vi "8742.vi"() -> ()   [LabVIEW 2012]
panel:
  out "Axis4 Mov":bool
  out "Axis3 Mov":bool
  out "Axis2 Mov":bool
  out "Axis1 Mov":bool
  out "Axis4 Pos":dbl
  out "Axis3 Pos":dbl
  out "Axis2 Pos":dbl
  out "Axis1 Pos":dbl
  in  "Axis4 set":dbl
  in  "Axis3 set":dbl
  in  "Axis2 set":dbl
  in  "Axis1 set":dbl
  in  "停止":bool
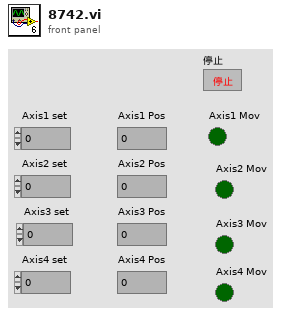
[diagram p1: front panel]
types:
  T1 = cluster{"CmdLib Out":refnum<k24>, "DeviceKey Out":string, "Device Address":i32}
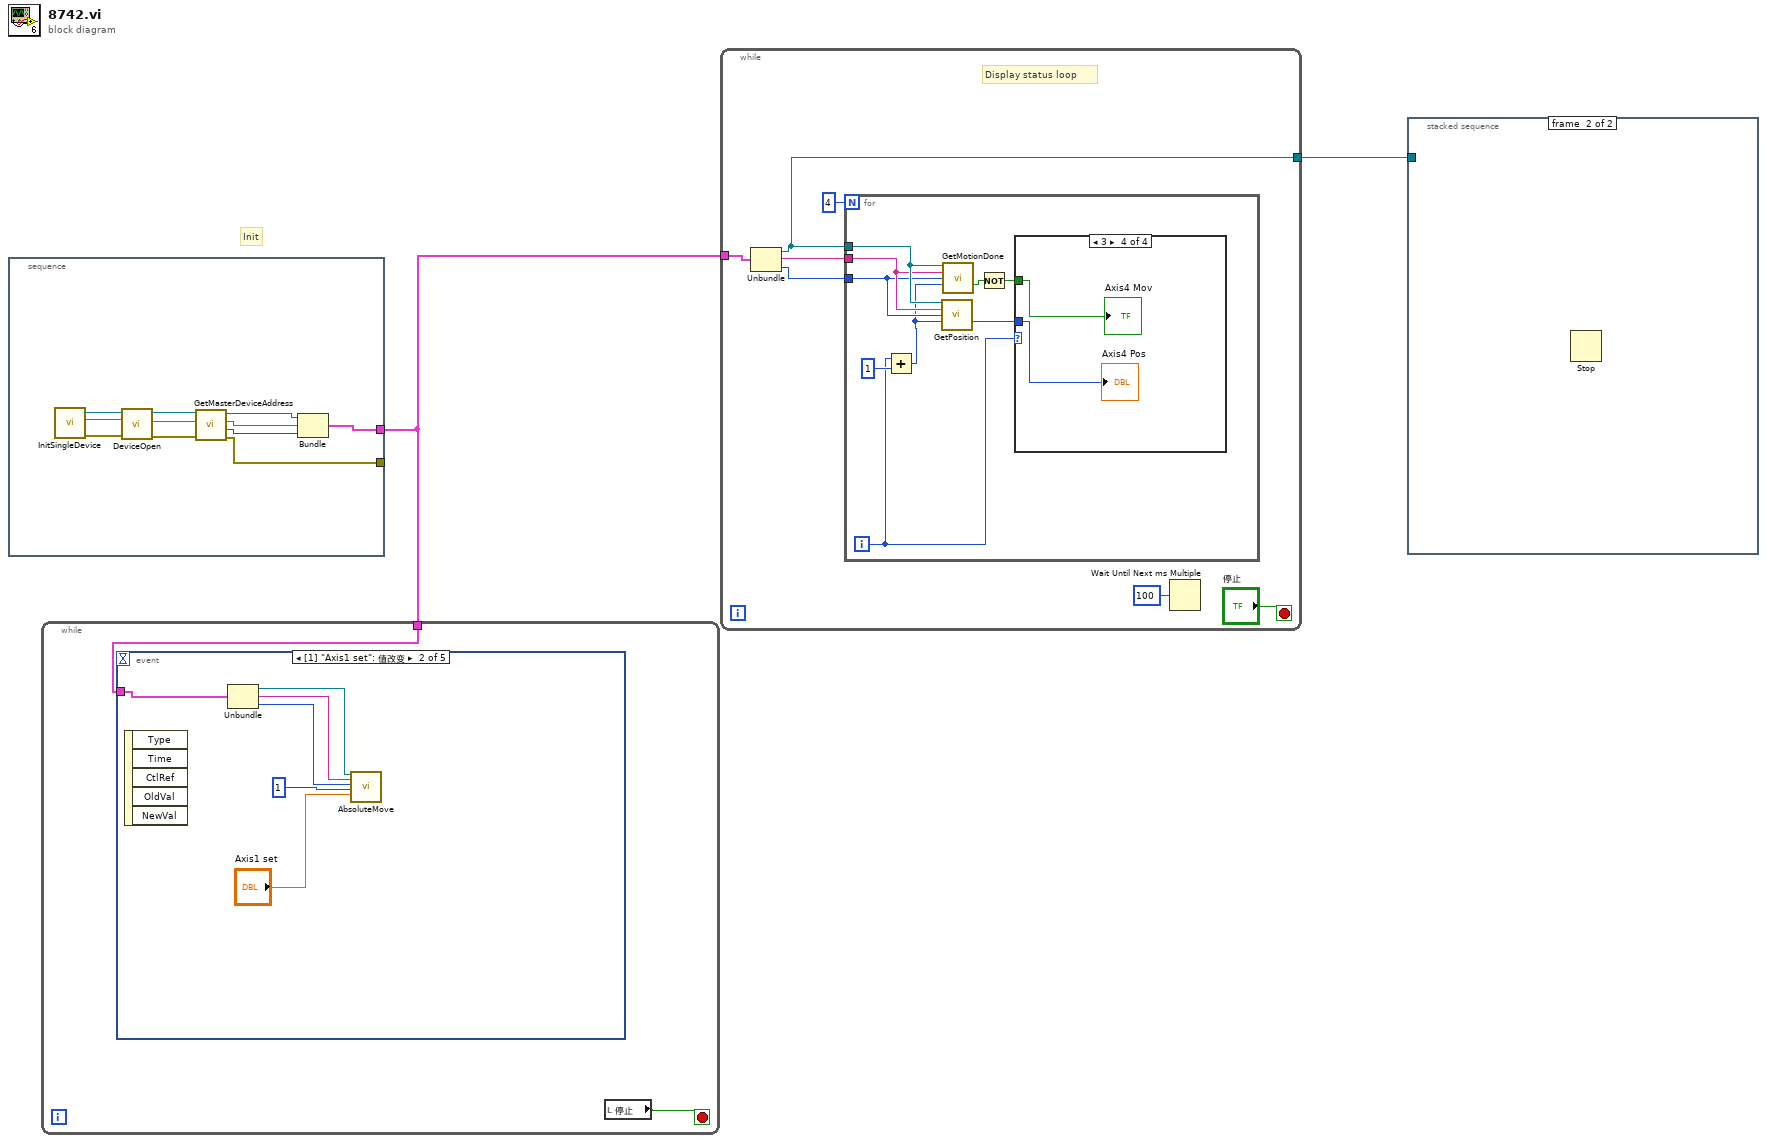
[diagram p0: block diagram]
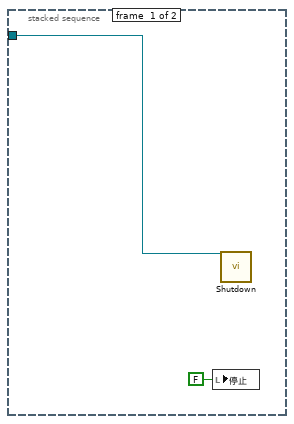
[diagram p2: hidden frame]
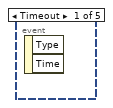
[diagram p3: hidden frame]
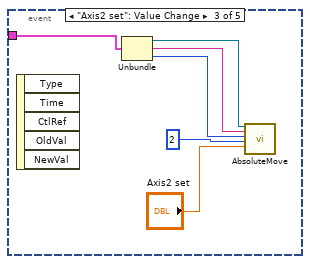
[diagram p4: hidden frame]
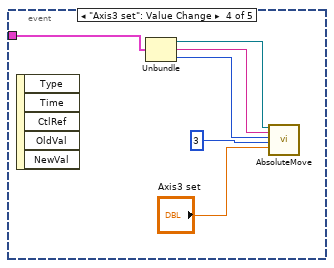
[diagram p5: hidden frame]
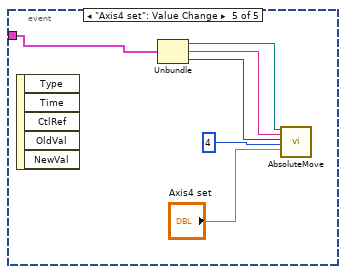
[diagram p6: hidden frame]
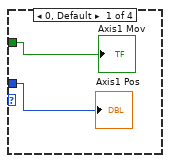
[diagram p7: hidden frame]
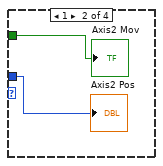
[diagram p8: hidden frame]
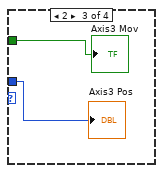
[diagram p9: hidden frame]
diagram:
  # "Init"
  n1 = stacked-sequence {
    tunnel: [w4] -> w2
    tunnel: [w3] -> _
    frame #0 {
      n2 = call "InitSingleDevice.vi"() -> ("error out"=w13:errorcluster, "DeviceKey Out"=w8:string, "CmdLib Out"=w9:refnum<k24>)  [unwired: 5 in]
      n3 = call "DeviceOpen.vi"("error in (no error)"=w13, "DeviceKey In"=w8, "CmdLib In"=w9) -> ("error out"=w12:errorcluster, "DeviceKey Out"=w11:string, "CmdLib Out"=w10:refnum<k24>)  [unwired: 2 in]
      n4 = call "GetMasterDeviceAddress.vi"("error in (no error)"=w12, "DeviceKey In"=w11, "CmdLib In"=w10) -> ("error out"=w3:errorcluster, "Device Address"=w5:i32, "DeviceKey Out"=w6:string, "CmdLib Out"=w7:refnum<k24>)  [unwired: 1 in]
      n5 = Bundle("CmdLib Out"=w7, "DeviceKey Out"=w6, "Device Address"=w5) -> (w4:T1)  [unwired: 1 in]
    }
  }
  n6 = while {
    tunnel: w2 -> [w15]
    stop <- w14 stop-if-true
    n7 = event shown="[1] \"Axis1 set\": 值改变" {
      selector: _ -> [_ _ _ _ _]
      dyn-events: _ -> [_ _ _ _ _]
      timeout: _ -> [_ _ _ _ _]
      tunnel: w15 -> [_ w21 w23 w29 w35]
      event Timeout {
        n8 = event-data() -> ()  [unwired: 1 in, 2 out]
      }
      event "Axis1 set": Value Change {
        n9 = event-data() -> ()  [unwired: 1 in, 5 out]
        n10 = Unbundle(w21) -> ("CmdLib Out"=w20:refnum<k24>, "DeviceKey Out"=w19:string, "Device Address"=w18:i32)
        n11 = call "AbsoluteMove.vi"("CmdLib In"=w20, "DeviceKey In"=w19, "Device Address In"=w18, "Motor"=1, "Target Pos"="Axis1 set") -> ()  [unwired: 11 in, 4 out]
      }
      event "Axis2 set": Value Change {
        n12 = event-data() -> ()  [unwired: 1 in, 5 out]
        n13 = Unbundle(w23) -> ("CmdLib Out"=w24:refnum<k24>, "DeviceKey Out"=w25:string, "Device Address"=w26:i32)
        n14 = call "AbsoluteMove.vi"("CmdLib In"=w24, "DeviceKey In"=w25, "Device Address In"=w26, "Motor"=2, "Target Pos"="Axis2 set") -> ()  [unwired: 11 in, 4 out]
      }
      event "Axis3 set": Value Change {
        n15 = event-data() -> ()  [unwired: 1 in, 5 out]
        n16 = Unbundle(w29) -> ("CmdLib Out"=w33:refnum<k24>, "DeviceKey Out"=w32:string, "Device Address"=w31:i32)
        n17 = call "AbsoluteMove.vi"("CmdLib In"=w33, "DeviceKey In"=w32, "Device Address In"=w31, "Motor"=3, "Target Pos"="Axis3 set") -> ()  [unwired: 11 in, 4 out]
      }
      event "Axis4 set": Value Change {
        n18 = event-data() -> ()  [unwired: 1 in, 5 out]
        n19 = Unbundle(w35) -> ("CmdLib Out"=w36:refnum<k24>, "DeviceKey Out"=w37:string, "Device Address"=w38:i32)
        n20 = call "AbsoluteMove.vi"("CmdLib In"=w36, "DeviceKey In"=w37, "Device Address In"=w38, "Motor"=4, "Target Pos"="Axis4 set") -> ()  [unwired: 11 in, 4 out]
      }
    }
    n21 = local read "停止"() -> (w14:bool)
  }
  n22 = while {
    tunnel: w2 -> [w45]
    tunnel: [w40] -> w1
    stop <- "停止" stop-if-true
    # "Display status loop"
    n23 = Unbundle(w45) -> ("CmdLib Out"=w40:refnum<k24>, "DeviceKey Out"=w44:string, "Device Address"=w43:i32)
    n24 = for {
      N: 4 -> [_]
      tunnel: w40 -> [w53]
      tunnel: w44 -> [w52]
      tunnel: w43 -> [w51]
      i -> [w47]
      n25 = Add(x=w47, y=1) -> (x+y=w50:i32)
      n26 = call "GetPosition.vi"("CmdLib In"=w53, "DeviceKey In"=w52, "Device Address In"=w51, "Motor"=w50) -> ("Position"=w54:i32)  [unwired: 7 in, 4 out]
      n27 = call "GetMotionDone.vi"("CmdLib In"=w53, "DeviceKey In"=w52, "Device Address In"=w51, "Motor"=w50) -> ("Is Motion Done"=w49:bool)  [unwired: 7 in, 4 out]
      n28 = Not(x=w49) -> (.not. x?=w48:bool)
      n29 = case shown="3" w47 {
        tunnel: w54 -> [w57 w59 w61 w63]
        tunnel: w48 -> [w56 w58 w60 w62]
        frame 0, Default {
          "Axis1 Pos" <- w57
          "Axis1 Mov" <- w56
        }
        frame 1 {
          "Axis2 Pos" <- w59
          "Axis2 Mov" <- w58
        }
        frame 2 {
          "Axis3 Pos" <- w61
          "Axis3 Mov" <- w60
        }
        frame 3 {
          "Axis4 Pos" <- w63
          "Axis4 Mov" <- w62
        }
      }
    }
    n30 = Wait Until Next ms Multiple(millisecond multiple=u32 100 ("毫秒倍数")) -> ()  [unwired: 1 out]
  }
  n31 = stacked-sequence {
    tunnel: w1 -> [w65 _]
    frame #0 {
      n32 = local write "停止"(FALSE ("停止")) -> ()
      n33 = call "Shutdown.vi"("CmdLib In"=w65) -> ()  [unwired: 5 in, 2 out]
    }
    frame #1 {
      n34 = Stop() -> ()  [unwired: 1 in]
    }
  }
